vi "StressDist_circ.vi"(7 "Corrigido":bool, 8 "Error In":errorcluster, 11 "main_FGV_data":T1={"pipe_properties"={"out_radius"=0.0, "in_radius"=0.0, "out_diameter"=0.0, "in_diameter"=0.0, "thickness"=0.0, "inertia"=0.0, "area"=0.0}, "DirPath"=path "L:/Documentos/00 SERVIÇOS/Tensão residual/Olapa 10-2017/Dados/Primeira Seção/Furos", "DirReport"=path "L:/Documentos/00 SERVIÇOS/Tensão residual/Olapa 10-2017/RelatóriosOlapa/Teste", "Points"=[], "ovalization_data"={"AngOval"=[0.0, 60.0, 120.0, 22.5, 45.0, 67.5, 90.0, 112.5, 135.0, 157.5, 180.0], "OvalDiam"=[324.25, 324.6, 324.55, 324.25, 324.55, 324.65, 324.6, 324.65, 324.55, 324.5, 324.4], "Plots"={"Ref"={"X"=[], "Y"=[]}, "Elipse"={"X"=[], "Y"=[]}, "Points"={"X"=[], "Y"=[]}}, "Ampliation"=100.0, "Results"={"MD"=0.0, "mD"=0.0, "Dmed"=0.0, "Oval"=0.0, "ang"=0.0, "X0"=0.0, "Y0"=0.0}, "fit"=[]}, "StressDist_data"={"Long"={"Plot"=[], "Fit"=[], "ColorMap"=[], "Data"=[], "peirce_data"={"Plot"=[], "Index removidos"=[]}}, "Circ"={"Plot"=[], "Fit"=[], "ColorMap"=[], "Data"=[], "peirce_data"={"Plot"=[], "Index removidos"=[]}}, "Shear"={"Plot"=[], "Fit"=[], "ColorMap"=[], "Data"=[], "peirce_data"={"Plot"=[], "Index removidos"=[]}}, "Equivalent"={"Plot"=[], "Fit"=[], "ColorMap"=[], "Data"=[], "peirce_data"={"Plot"=[], "Index removidos"=[]}}}, "pressure_data"={"Pressure"=[], "StressCircOval"=[], "StressCirc"=[], "StressLong"=[], "Plot"=[], "Angle"=[]}, "Reload"=FALSE}) -> (0 "Error Out":errorcluster, 3 "main_FGV_data-out":T1={"pipe_properties"={"out_radius"=0.0, "in_radius"=0.0, "out_diameter"=0.0, "in_diameter"=0.0, "thickness"=0.0, "inertia"=0.0, "area"=0.0}, "DirPath"=path "L:/Documentos/00 SERVIÇOS/Tensão residual/Olapa 10-2017/Dados/Primeira Seção/Furos", "DirReport"=path "L:/Documentos/00 SERVIÇOS/Tensão residual/Olapa 10-2017/RelatóriosOlapa/Teste", "Points"=[], "ovalization_data"={"AngOval"=[0.0, 60.0, 120.0, 22.5, 45.0, 67.5, 90.0, 112.5, 135.0, 157.5, 180.0], "OvalDiam"=[324.25, 324.6, 324.55, 324.25, 324.55, 324.65, 324.6, 324.65, 324.55, 324.5, 324.4], "Plots"={"Ref"={"X"=[], "Y"=[]}, "Elipse"={"X"=[], "Y"=[]}, "Points"={"X"=[], "Y"=[]}}, "Ampliation"=100.0, "Results"={"MD"=0.0, "mD"=0.0, "Dmed"=0.0, "Oval"=0.0, "ang"=0.0, "X0"=0.0, "Y0"=0.0}, "fit"=[]}, "StressDist_data"={"Long"={"Plot"=[], "Fit"=[], "ColorMap"=[], "Data"=[], "peirce_data"={"Plot"=[], "Index removidos"=[]}}, "Circ"={"Plot"=[], "Fit"=[], "ColorMap"=[], "Data"=[], "peirce_data"={"Plot"=[], "Index removidos"=[]}}, "Shear"={"Plot"=[], "Fit"=[], "ColorMap"=[], "Data"=[], "peirce_data"={"Plot"=[], "Index removidos"=[]}}, "Equivalent"={"Plot"=[], "Fit"=[], "ColorMap"=[], "Data"=[], "peirce_data"={"Plot"=[], "Index removidos"=[]}}}, "pressure_data"={"Pressure"=[], "StressCircOval"=[], "StressCirc"=[], "StressLong"=[], "Plot"=[], "Angle"=[]}, "Reload"=FALSE})   [LabVIEW 2016]
uses:
  MainFGV/main_FGV_data.ctl
  MainFGV/pipe_properties.ctl
  StressCalculations/point_data.ctl
  Ovalization/ovalization_data.ctl
  StressDist_data.ctl
  StressDist_single_data.ctl
  Peirce/peirce_data.ctl
  Pressure/pressure_data.ctl
  StressDist_types.ctl
  Report/report_mods.ctl
  ExternalDependencies/AlgenLabVIEW/Code/TypeDefs/termination_data.ctl
  ExternalDependencies/AlgenLabVIEW/Code/TypeDefs/basic_config.ctl
panel:
  out "CircStressCM":dbl[][](graph)
  out "CircStress":cluster{"X":dbl[], "Y":dbl[]}[](graph) caption="Ovalização"
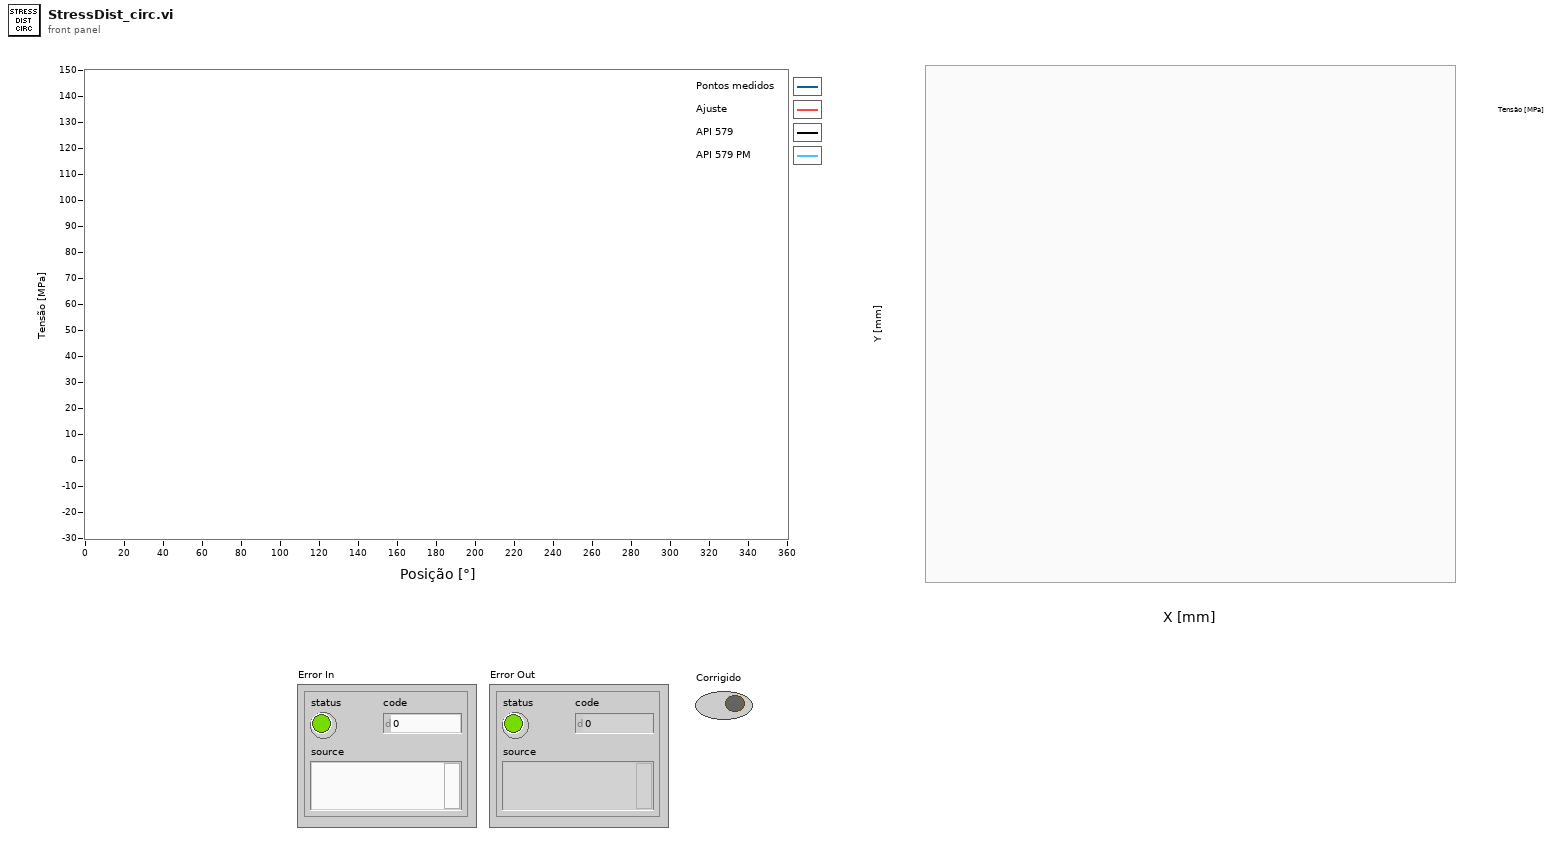
[diagram p1: front panel]
types:
  T1 = typedef "main_FGV_data.ctl" = cluster{"pipe_properties":T2, "DirPath":path, "DirReport":path, "Points":T3[], "ovalization_data":T4, "StressDist_data":T5, "pressure_data":T8, "Reload":bool}
  T2 = typedef "pipe_properties.ctl" = cluster{"out_radius":dbl, "in_radius":dbl, "out_diameter":dbl, "in_diameter":dbl, "thickness":dbl, "inertia":dbl, "area":dbl}
  T3 = typedef "point_data.ctl" = cluster{"LongStress":dbl, "CircStress":dbl, "ShearStress":dbl, "Pressure":dbl, "Angle":dbl, "Thickness":dbl, "HoleDiam":dbl, "EquiStress":dbl, "S1":dbl, "S2":dbl, "Beta":dbl}
  T4 = typedef "ovalization_data.ctl" = cluster{"AngOval":dbl[], "OvalDiam":dbl[], "Plots":cluster{"Ref":cluster{"X":dbl[], "Y":dbl[]}, "Elipse":cluster{"X":dbl[], "Y":dbl[]}, "Points":cluster{"X":dbl[], "Y":dbl[]}}, "Ampliation":dbl, "Results":cluster{"MD":dbl, "mD":dbl, "Dmed":dbl, "Oval":dbl, "ang":dbl, "X0":dbl, "Y0":dbl}, "fit":dbl[]}
  T5 = typedef "StressDist_data.ctl" = cluster{"Long":T6, "Circ":T6, "Shear":T6, "Equivalent":T6}
  T6 = typedef "StressDist_single_data.ctl" = cluster{"Plot":cluster{"Angle":dbl[], "Stress":dbl[]}[], "Fit":dbl[], "ColorMap":dbl[][], "Data":string[][], "peirce_data":T7}
  T7 = typedef "peirce_data.ctl" = cluster{"Plot":cluster{"Array":dbl[], "Array":dbl[]}[], "Index removidos":i32[]}
  T8 = typedef "pressure_data.ctl" = cluster{"Pressure":dbl[], "StressCircOval":dbl[], "StressCirc":dbl[], "StressLong":dbl[], "Plot":cluster{"Angle":dbl[], "Stress":dbl[]}[], "Angle":dbl[]}
  T9 = typedef "report_mods.ctl" = enum16{"Init", "Table", "Graph", "TablefromGraph", "End"}
  T10 = typedef "StressDist_types.ctl" = enum16{"Long", "Circ", "Shear", "Equivalent"}
  T11 = typedef "basic_config.ctl" = cluster{"parameters_range":cluster{"Max":dbl, "Min":dbl}[], "Initial elements":i32}
  T12 = typedef "termination_data.ctl" = cluster{"MaxGen":cluster{"Generations":i32, "Active":bool}, "CostFunctionTol":cluster{"Tol":dbl, "Active":bool}, "GensEstab":cluster{"Generations":i32, "Active":bool}}
  T13 = typedef "GenAlg_data.ctl" = cluster{"BasicCondfig":T11, "elements":T14[], "CostFunction":refnum<vi>, "GenerationData":T15, "SelectionData":T16, "SimulatedAnnealingData":T17, "CostFunctionData":variant, "MultiEval_data":T18, "TerminationData":T12}
  T14 = typedef "element.ctl" = cluster{"Parameters":dbl[], "Cost":dbl}
  T15 = typedef "geration_data.ctl" = cluster{"ElementsCreated":i32}
  T16 = typedef "selection_data.ctl" = cluster{"ElementsSelected":i32}
  T17 = typedef "SimulatedAnnealing_data.ctl" = cluster{"AnnealingFactor":dbl, "Active":bool}
  T18 = typedef "multi_eval_data.ctl" = cluster{"Active":bool, "MultiEvalFunction":refnum<vi>}
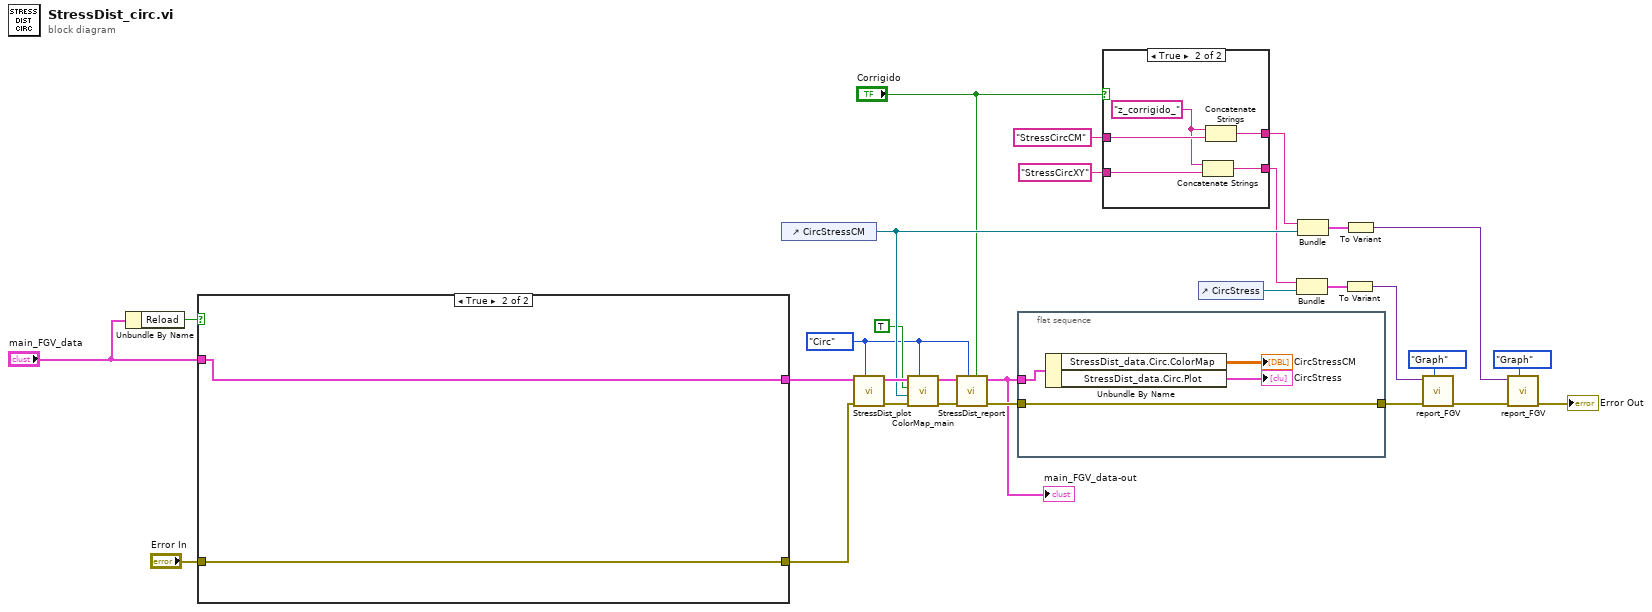
[diagram p0: block diagram]
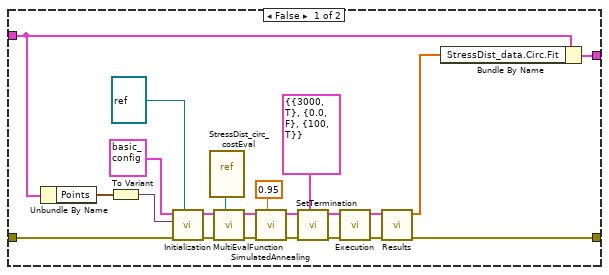
[diagram p3: hidden frame]
diagram:
  w5 = StressDist_types."Circ" ("StressDist_types")
  n1 = Unbundle By Name("main_FGV_data") -> ("Reload"=w2:bool)
  n2 = case shown="True" w2 {
    tunnel: [w34 w52] -> w29
    tunnel: [w32 w53] -> w23
    tunnel: "main_FGV_data" -> [w31 w53]
    tunnel: "Error In" -> [w30 w52]
    frame False {
      n3 = Unbundle By Name(w31) -> ("Points"=w39:T3[])
      n4 = To Variant(anything=w39) -> (Variant=w38:variant)
      n5 = call "Initialization.vi"("CostFunction"=refnum<vi> refnum, "Error In"=w30, "CostFunctionData"=w38, "basic_config"=T11 {"parameters_range"=[{"Max"=10000.0, "Min"=-10000.0}, {"Max"=10000.0, "Min"=-10000.0}, {"Max"=10000.0, "Min"=-10000.0}], "Initial elements"=20}) -> ("Error Out"=w50:errorcluster, "GenAlg_data"=w51:T13)  [unwired: 6 in]
      n6 = vi-ref "StressDist_circ_costEval.vi"() -> (w35:refnum<vi>)
      n7 = call "MultiEvalFunction.vi"("MultiEvalFunction"=w35, "Error In"=w50, "GenAlg_data"=w51) -> ("Error Out"=w49:errorcluster, "GenAlg_data-out"=w45:T13)  [unwired: 7 in]
      n8 = call "SimulatedAnnealing.vi"("AnnealingFactor"=0.95, "Error In"=w49, "GenAlg_data"=w45) -> ("Error Out"=w48:errorcluster, "GenAlg_data-out"=w44:T13)  [unwired: 7 in]
      n9 = call "SetTermination.vi"("TerminationData"=T12 {"MaxGen"={"Generations"=3000, "Active"=TRUE}, "CostFunctionTol"={"Tol"=0.0, "Active"=FALSE}, "GensEstab"={"Generations"=100, "Active"=TRUE}}, "Error In"=w48, "GenAlg_data"=w44) -> ("Error Out"=w47:errorcluster, "GenAlg_data-out"=w43:T13)  [unwired: 7 in]
      n10 = call "Execution.vi"("Error In"=w47, "GenAlg_data"=w43) -> ("Error Out"=w46:errorcluster, "GenAlg_data-out"=w42:T13)  [unwired: 8 in]
      n11 = call "Results.vi"("Error In"=w46, "GenAlg_data"=w42) -> ("Error Out"=w34:errorcluster, "MinPoint"=w33:dbl[])  [unwired: 7 in, 1 out]
      n12 = Bundle By Name(cluster=w31, "StressDist_data.Circ.Fit"=w33) -> (w32:T1)
    }
    frame True {
    }
  }
  n13 = control-ref of="CircStressCM"() -> (w15:refnum<vi>)
  n14 = call "StressDist_plot.vi"("StressDist_types"=w5, "Error In"=w29, "main_FGV_data"=w23) -> ("Error Out"=w22:errorcluster, "main_FGV_data-out"=w21:T1)  [unwired: 7 in]
  n15 = call "ColorMap_main.vi"("StressDist_types"=w5, "Error In"=w22, "RefCM"=w15, "Deformed"=TRUE, "main_FGV_data"=w21) -> ("Error Out"=w9:errorcluster, "main_FGV_data-out"=w7:T1)  [unwired: 5 in]
  n16 = call "StressDist_report.vi"("Corrigido"="Corrigido", "StressDist_types"=w5, "Error In"=w9, "main_FGV_data"=w7) -> ("Error Out"=w8:errorcluster, "main_FGV_data-out"=w6:T1)  [unwired: 6 in]
  "main_FGV_data-out" <- w6
  n17 = flat-sequence {
    tunnel: w6 -> [w57]
    tunnel: w8 -> [w55]
    tunnel: [w55] -> w27
    frame #0 {
      n18 = Unbundle By Name(w57) -> ("StressDist_data.Circ.ColorMap"=→"CircStressCM":dbl[][], "StressDist_data.Circ.Plot"=→"CircStress":cluster{"Angle":dbl[], "Stress":dbl[]}[])
    }
  }
  n19 = case shown="True" "Corrigido" {
    tunnel: "StressCircCM" -> [w59 w64]
    tunnel: "StressCircXY" -> [w58 w62]
    tunnel: [w59 w63] -> w11
    tunnel: [w58 w61] -> w10
    frame False {
    }
    frame True {
      w60 = "z_corrigido_" ("string")
      n20 = Concatenate Strings(w60, w62) -> (w61:string)
      n21 = Concatenate Strings(w60, w64) -> (w63:string)
    }
  }
  n22 = control-ref of="CircStress"() -> (w24:refnum<vi>)
  n23 = Bundle(w10, "CircStress"=w24) -> (w26:cluster{string, "CircStress":refnum<vi>})  [unwired: 1 in]
  n24 = Bundle(w11, "CircStressCM"=w15) -> (w17:cluster{string, "CircStressCM":refnum<vi>})  [unwired: 1 in]
  n25 = To Variant(anything=w26) -> (Variant=w25:variant)
  n26 = To Variant(anything=w17) -> (Variant=w16:variant)
  n27 = call "report_FGV.vi"("report_mods"=report_mods."Graph", "Error In"=w27, "Data in"=w25) -> ("Error Out"=w19:errorcluster)  [unwired: 8 in]
  n28 = call "report_FGV.vi"("report_mods"=report_mods."Graph", "Error In"=w19, "Data in"=w16) -> ("Error Out"=→"Error Out":errorcluster)  [unwired: 8 in]
